vi "Write Command Response.vi"(8 "error in (no error)":errorcluster, 10 "Command Response":string, 11 "ESM303 in":refnum<class "ESM303.lvclass">) -> (0 "error out":errorcluster, 3 "ESM303 out":refnum<class "ESM303.lvclass">)   [LabVIEW 2018, in "ESM303.lvlib" / "ESM303.lvclass"]
uses:
  ESM303.lvclass
  ESM303.lvclass/ESM303.ctl
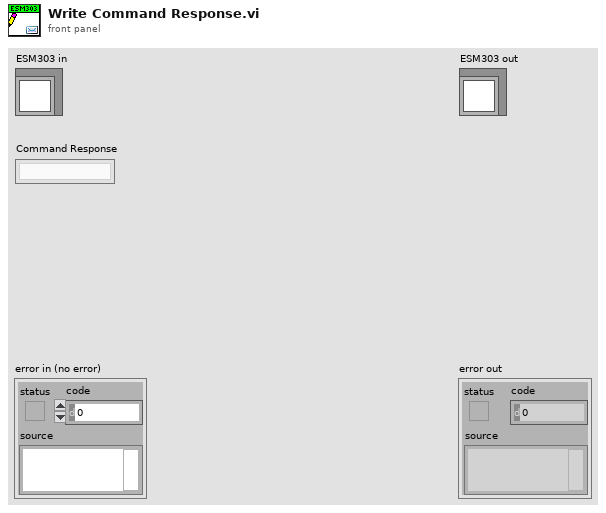
[diagram p1: front panel]
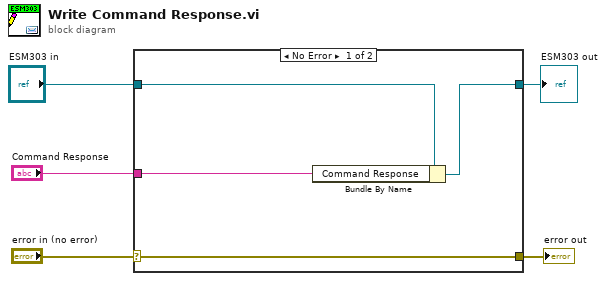
[diagram p0: block diagram]
diagram:
  n1 = case shown="No Error" "error in (no error)" {
    selector: "error in (no error)" -> [w9 w10]
    tunnel: [w9 w10] -> w4
    tunnel: [w7 w11] -> w2
    tunnel: "ESM303 in" -> [w8 w11]
    tunnel: "Command Response" -> [w6 _]
    frame No Error {
      n2 = Bundle By Name(cluster=w8, "Command Response"=w6) -> (w7:refnum<class "ESM303.lvclass">)
    }
    frame Error {
    }
  }
  "error out" <- w4
  "ESM303 out" <- w2
